vi "PointerArray_Delete Pointer.vi"(8 "Error":errorcluster, 9 "Name":string, 10 "Index":i32=-1, 11 "Pointer Array":refnum<class "((Pointer)).lvclass">[](array[class])) -> (0 "Error Out":errorcluster, 1 "Pointer Out":refnum<class "((Pointer)).lvclass">, 2 "Index Out":i32, 3 "Pointer Array Out":refnum<class "((Pointer)).lvclass">[](array[class]), 4 "Found Out":bool)   [LabVIEW 2016, in "(WavBuf).lvclass"]
uses:
  WavBuf/(WavBuf).lvclass
  Pointer/((Pointer)).lvclass
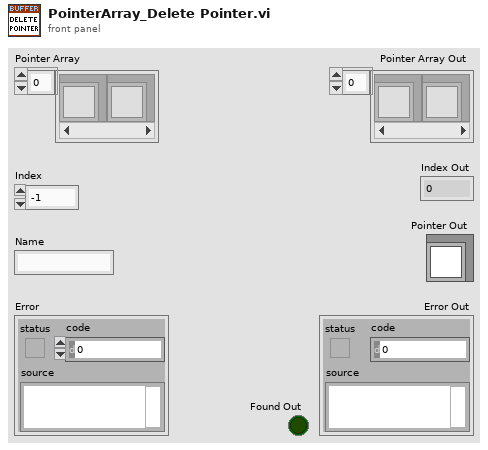
[diagram p1: front panel]
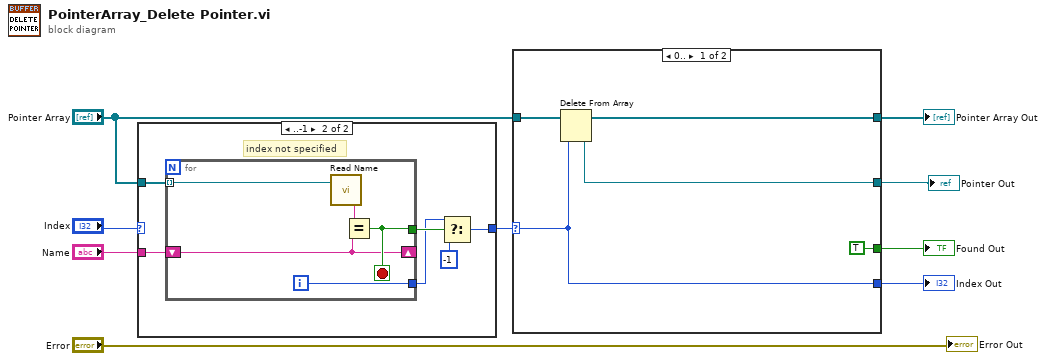
[diagram p0: block diagram]
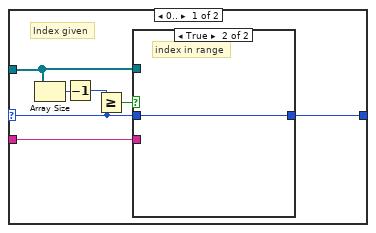
[diagram p2: hidden frame]
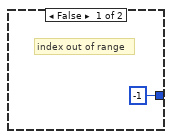
[diagram p3: hidden frame]
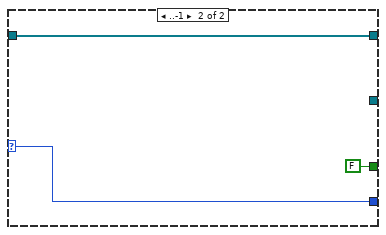
[diagram p4: hidden frame]
diagram:
  n1 = case shown="..-1" "Index" {
    selector: "Index" -> [w12 _]
    tunnel: "Name" -> [w10 w24]
    tunnel: "Pointer Array" -> [w15 w23]
    tunnel: [w11 w21] -> w1
    frame 0.. {
      # "Index given"
      n2 = Array Size(array=w15) -> (size(s)=w16:i32)
      n3 = Decrement(x=w16) -> (x-1=w14:i32)
      n4 = Greater Or Equal?(x=w14, y=w12) -> (x >= y?=w13:bool)
      n5 = case shown="True" w13 {
        tunnel: w15 -> [_ _]
        tunnel: w12 -> [_ w18]
        tunnel: [-1 ("Index") w18] -> w11
        tunnel: w10 -> [_ _]
        frame False {
          # "index out of range"
        }
        frame True {
          # "index in range"
        }
      }
    }
    frame ..-1 {
      # "index not specified"
      n6 = for {
        tunnel: w23 -> [w25] mode=indexing
        tunnel: [w28] -> w22
        tunnel: [w27] -> w20
        shift-right: [w26] -> _
        shift-left: w24 -> [w26]
        i -> [w27]
        stop <- w28 stop-if-true
        n7 = call "Read Name.vi"("((Pointer))"=w25) -> ("Name Out"=w29:string)  [unwired: 2 in]
        n8 = Equal?(x=w29, y=w26) -> (x = y?=w28:bool)
      }
      n9 = Select(t=w20, s=w22, f=-1) -> (s? t:f=w21:i32)
    }
  }
  n10 = case shown="0.." w1 {
    selector: w1 -> [w30 w35]
    tunnel: "Pointer Array" -> [w33 w37]
    tunnel: [w30 w35] -> w6
    tunnel: [TRUE FALSE] -> w5
    tunnel: [w31 _] -> w4
    tunnel: [w32 w37] -> w3
    frame 0.. {
      n11 = Delete From Array(array=w33, index=w30) -> (deleted portion=w31:refnum<class "((Pointer)).lvclass">, array with subset deleted=w32:refnum<class "((Pointer)).lvclass">[])  [unwired: 1 in]
    }
    frame ..-1 {
    }
  }
  "Pointer Out" <- w4
  "Pointer Array Out" <- w3
  "Index Out" <- w6
  "Found Out" <- w5
  "Error Out" <- "Error"
